vi "TemperatureHumidityMonitor.vi"() -> ()   [LabVIEW 2013]
uses:
  InstrControl/ArduinoControl/ArduinoControl.lvclass
  InstrControl/InstrumentSetup.vi
  InstrControl/InstrControl.lvclass
panel:
  in  "VISA address":refnum<visa-resource-name>="COM24"
  in  "Duration":u32=43200 step=3600 format="%<%H:%M:%S>t"
  in  "Run":bool
  in  "quit":bool
  out "Run time":u32 format="%<%H:%M:%S>t"
  out "Humidity":dbl caption="Humidity [%]"
  out "Temp.":dbl caption="Temp. [°C]"
  in  "Interval [s]":u32=10
  out "Tgraph":cluster{u32[], dbl[]}[](graph)
  # "Temperature & Humidity Monitor"
  # "University of\nCambridge"
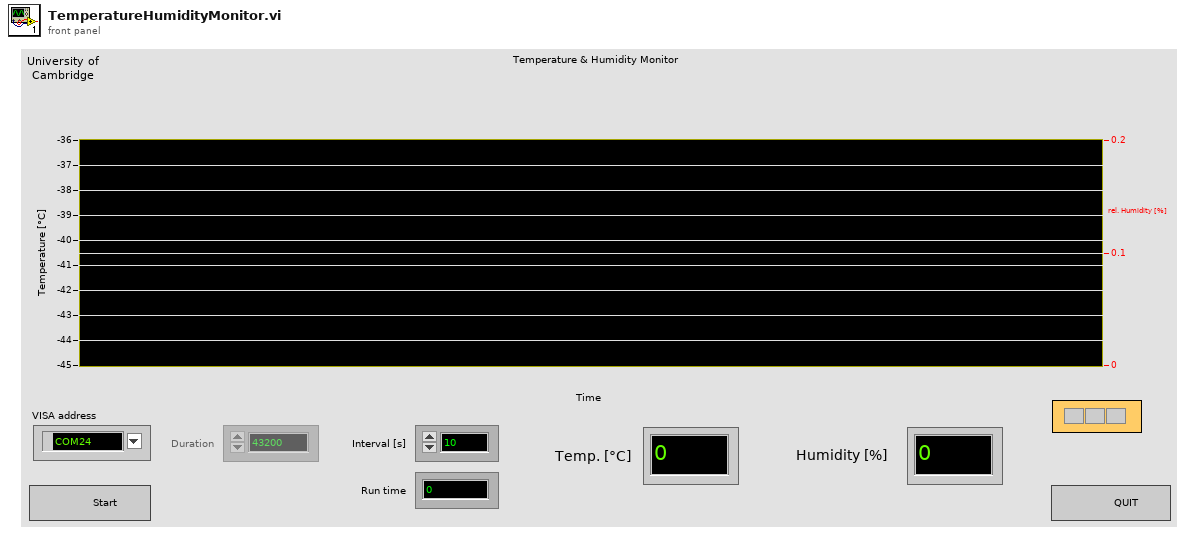
[diagram p1: front panel]
types:
  T1 = cluster{"VISA address":refnum<visa-resource-name>, "T sensor":enum16{"SHT", "DS"}, "Arduino":refnum<class "ArduinoControl.lvclass">}
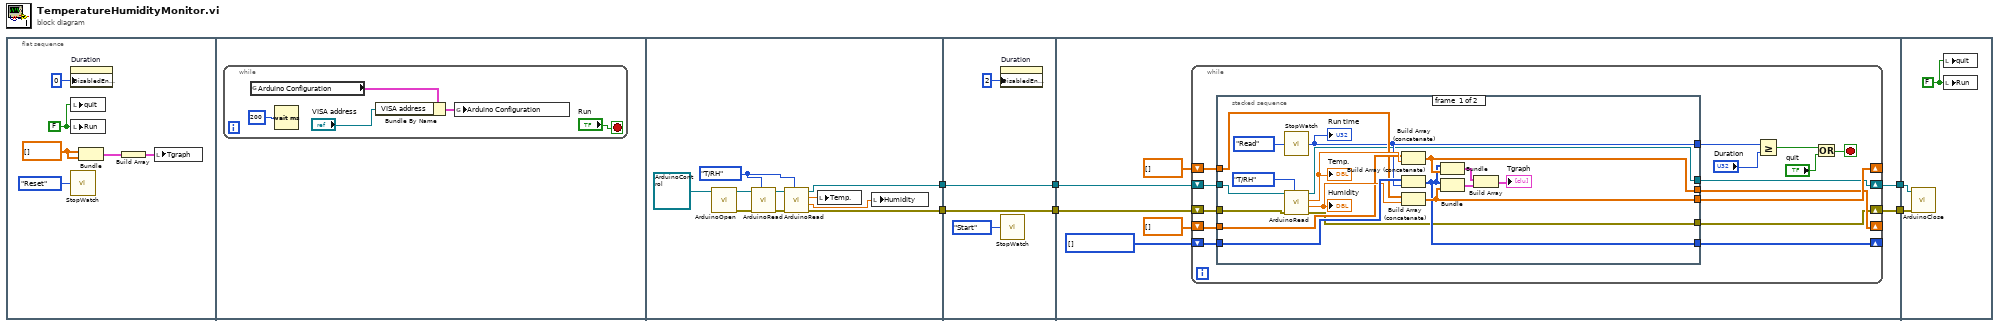
[diagram p0: block diagram]
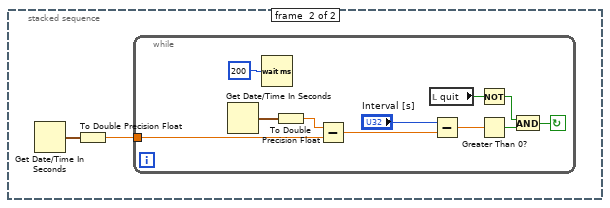
[diagram p2: hidden frame]
diagram:
  n1 = flat-sequence {
    tunnel: [w24] -> w5
    tunnel: [w23] -> w2
    tunnel: [w29] -> w6
    tunnel: w5 -> [w29]
    tunnel: [w28] -> w3
    tunnel: w2 -> [w28]
    tunnel: w6 -> [w35]
    tunnel: [w34] -> w4
    tunnel: w3 -> [w33]
    tunnel: [w32] -> w1
    tunnel: w4 -> [w86]
    tunnel: w1 -> [w85]
    frame #0 {
      w10 = dbl[] []
      w11 = FALSE
      n2 = property on="Duration" class="DigNum (strict)"("DisabledEnum"=0) -> ()  [unwired: 2 in, 2 out]
      n3 = local write "quit"(w11) -> ()
      n4 = local write "Run"(w11) -> ()
      n5 = call "StopWatch.vi"("Action"=enum16{"Start", "Stop", "Read", "Reset"}."Reset") -> ()  [unwired: 5 out]
      n6 = Bundle(w10, w10) -> (w8:cluster{dbl[], dbl[]})  [unwired: 1 in]
      n7 = Build Array(w8) -> (w9:cluster{dbl[], dbl[]}[])
      n8 = local write "Tgraph"(w9) -> ()
    }
    frame #1 {
      n9 = while {
        stop <- "Run" stop-if-true
        n10 = global read "InstrumentSetup.vi" "Arduino Configuration"() -> (w13:T1)
        n11 = Wait (ms)(milliseconds to wait=u32 200) -> ()  [unwired: 1 out]
        n12 = Bundle By Name(cluster=w13, "VISA address"="VISA address") -> (w15:T1)
        n13 = global write "InstrumentSetup.vi" "Arduino Configuration"(w15) -> ()
      }
    }
    frame #2 {
      w18 = enum16{"T/RH", "Interlock", "Edgesense"}."T/RH" ("Arduino function")
      n14 = call "ArduinoOpen.vi"("ArduinoControl in"=refnum<class "ArduinoControl.lvclass"> refnum) -> ("error out"=w22:errorcluster, "ArduinoControl out"=w21:refnum<class "ArduinoControl.lvclass">)  [unwired: 9 in]
      n15 = call "ArduinoRead.vi"("Arduino function"=w18, "error in (no error)"=w22, "ArduinoControl in"=w21) -> ("error out"=w19:errorcluster, "ArduinoControl out"=w20:refnum<class "ArduinoControl.lvclass">)  [unwired: 3 in, 4 out]
      n16 = call "ArduinoRead.vi"("Arduino function"=w18, "error in (no error)"=w19, "ArduinoControl in"=w20) -> ("error out"=w23:errorcluster, "rel. Humidity [%]"=w27:dbl, "Temperature [°C]"=w26:dbl, "ArduinoControl out"=w24:refnum<class "ArduinoControl.lvclass">)  [unwired: 3 in, 2 out]
      n17 = local write "Temp."(w26) -> ()
      n18 = local write "Humidity"(w27) -> ()
    }
    frame #3 {
      n19 = property on="Duration" class="DigNum (strict)"("DisabledEnum"=2) -> ()  [unwired: 2 in, 2 out]
      n20 = call "StopWatch.vi"("Action"=enum16{"Start", "Stop", "Read", "Reset"}."Start") -> ()  [unwired: 5 out]
    }
    frame #4 {
      n21 = while {
        shift-right: [w48] -> _
        shift-left: u32[] [] -> [w49]
        shift-right: [w44] -> _
        shift-left: dbl[] [] -> [w47]
        shift-right: [w45] -> _
        shift-left: dbl[] [] -> [w46]
        shift-right: [w41] -> w34
        shift-left: w35 -> [w42]
        shift-right: [w39] -> w32
        shift-left: w33 -> [w40]
        stop <- w50 stop-if-true
        n22 = stacked-sequence {
          tunnel: w49 -> [w70 _]
          tunnel: [w63 _] -> w48
          tunnel: w47 -> [w67 _]
          tunnel: w46 -> [w66 _]
          tunnel: [w65 _] -> w45
          tunnel: [w64 _] -> w44
          tunnel: [w59 _] -> w43
          tunnel: w42 -> [w58 _]
          tunnel: [w57 _] -> w41
          tunnel: w40 -> [w56 _]
          tunnel: [w55 _] -> w39
          frame #0 {
            n23 = call "StopWatch.vi"("Action"=enum16{"Start", "Stop", "Read", "Reset"}."Read") -> ("Time elapsed"=w59:u32)  [unwired: 4 out]
            "Run time" <- w59
            n24 = call "ArduinoRead.vi"("Arduino function"=enum16{"T/RH", "Interlock", "Edgesense"}."T/RH", "error in (no error)"=w56, "ArduinoControl in"=w58) -> ("error out"=w55:errorcluster, "rel. Humidity [%]"=w69:dbl, "Temperature [°C]"=w68:dbl, "ArduinoControl out"=w57:refnum<class "ArduinoControl.lvclass">)  [unwired: 3 in, 2 out]
            "Humidity" <- w69
            "Temp." <- w68
            n25 = Build Array (concatenate)(w67, w68) -> (w64:dbl[])
            n26 = Build Array (concatenate)(w70, w59) -> (w63:u32[])
            n27 = Build Array (concatenate)(w66, w69) -> (w65:dbl[])
            n28 = Bundle(w63, w64) -> (w62:cluster{u32[], dbl[]})  [unwired: 1 in]
            n29 = Bundle(w63, w65) -> (w61:cluster{u32[], dbl[]})  [unwired: 1 in]
            n30 = Build Array(w62, w61) -> (→"Tgraph":cluster{u32[], dbl[]}[])
          }
          frame #1 {
            n31 = Get Date/Time In Seconds() -> (seconds since 1Jan1904=w73:timestamp)
            n32 = To Double Precision Float(number=w73) -> (double precision float=w72:dbl)
            n33 = while {
              tunnel: w72 -> [w81]
              stop <- w74 continue-if-true
              n34 = Get Date/Time In Seconds() -> (seconds since 1Jan1904=w83:timestamp)
              n35 = Wait (ms)(milliseconds to wait=u32 200) -> ()  [unwired: 1 out]
              n36 = To Double Precision Float(number=w83) -> (double precision float=w82:dbl)
              n37 = Subtract(x=w82, y=w81) -> (x-y=w80:dbl)
              n38 = local read "quit"() -> (w77:bool)
              n39 = Subtract(x="Interval [s]", y=w80) -> (x-y=w78:dbl)
              n40 = Not(x=w77) -> (.not. x?=w76:bool)
              n41 = Greater Than 0?(x=w78) -> (x > 0?=w75:bool)
              n42 = And(x=w76, y=w75) -> (x .and. y?=w74:bool)
            }
          }
        }
        n43 = Greater Or Equal?(x=w43, y="Duration") -> (x >= y?=w51:bool)
        n44 = Or(x=w51, y="quit") -> (x .or. y?=w50:bool)
      }
    }
    frame #5 {
      w87 = FALSE
      n45 = call "ArduinoClose.vi"("error in (no error)"=w85, "ArduinoControl in"=w86) -> ()  [unwired: 8 in, 2 out]
      n46 = local write "quit"(w87) -> ()
      n47 = local write "Run"(w87) -> ()
    }
  }
